vi "Enrichment Chamber.vi"(7 "Speed Upgrades":u32 max=8) -> (0 "Yellow Cake/s":ext, 1 "Uranium Ingots/s":ext, 2 "Yellow Cake/t":ext, 3 "Uranium Ingots/t":ext)   [LabVIEW 2023]
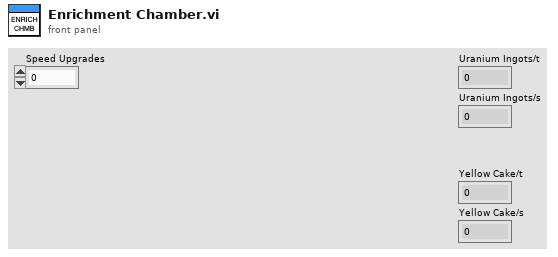
[diagram p1: front panel]
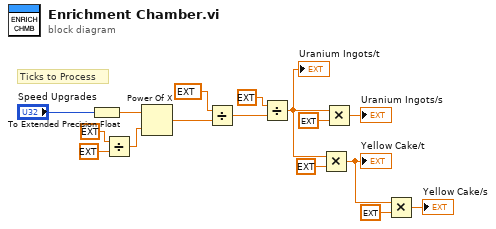
[diagram p0: block diagram]
diagram:
  # "Ticks to Process"
  n1 = To Extended Precision Float(1:"Speed Upgrades") -> (0:w3:ext)
  n2 = Divide(x=ext 4.0, y=ext 3.0) -> (x/y=w4:ext)
  n3 = Power Of X(1:w4, 2:w3) -> (0:w1:ext)
  n4 = Divide(x=ext 200.0 ("y"), y=w1) -> (x/y=w12:ext)
  n5 = Divide(x=ext 1.0, y=w12) -> (x/y=w9:ext)
  "Uranium Ingots/t" <- w9
  n6 = Multiply(x=w9, y=ext 2.0) -> (x*y=w7:ext)
  "Yellow Cake/t" <- w7
  n7 = Multiply(x=w9, y=ext 20.0) -> (x*y=→"Uranium Ingots/s":ext)
  n8 = Multiply(x=w7, y=ext 20.0) -> (x*y=→"Yellow Cake/s":ext)
